vi "sub_psk_symbol_map_gen.vi"(9 "Gray code?":bool=TRUE, 11 "M-PSK":i32=4) -> (1 "index map":u32[](array[numeric]), 3 "symbol map":cdb[](array[numeric]))   [LabVIEW 2014]
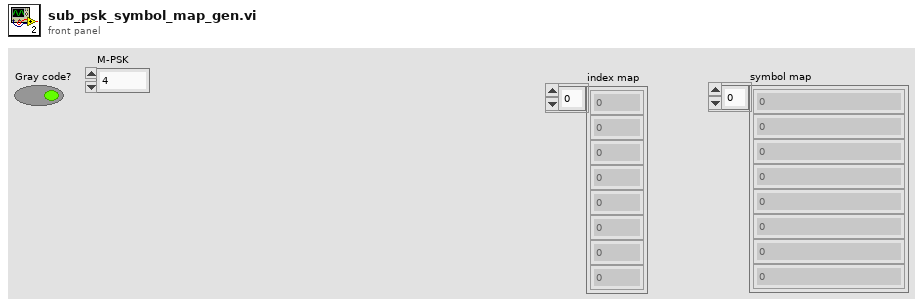
[diagram p1: front panel]
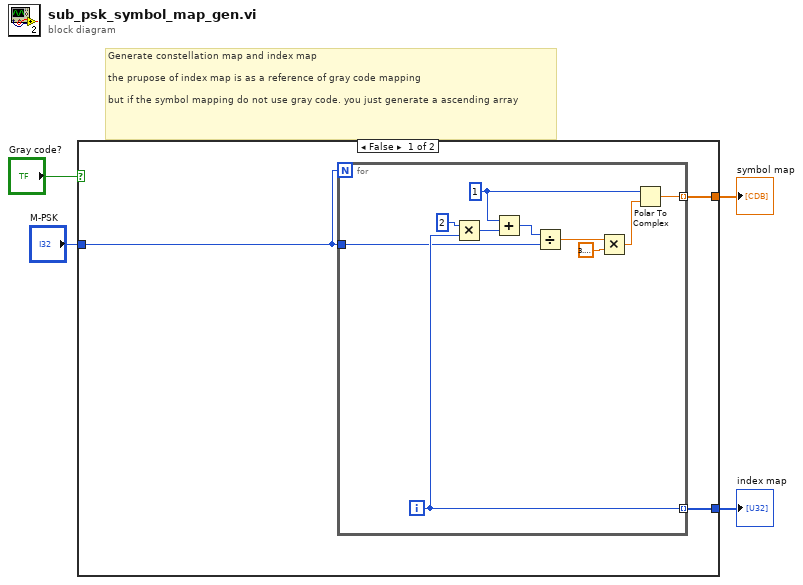
[diagram p0: block diagram]
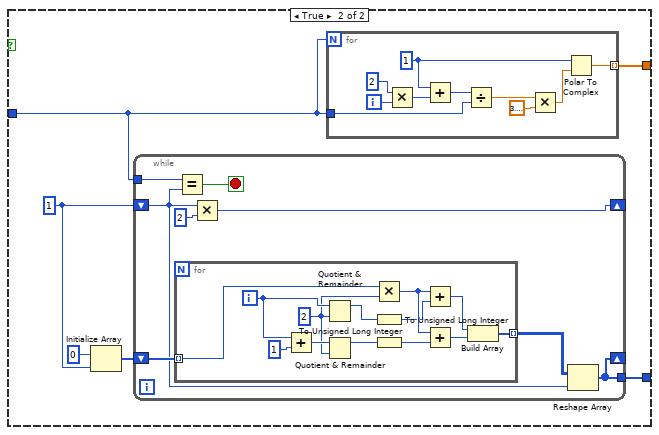
[diagram p2: hidden frame]
diagram:
  # "Generate constellation map and index map\n\nthe prupose of index map is as a reference of gray code mapping\n\nbut if the symbol mapping do not use gray code. you just generate a ascending array"
  n1 = case shown="False" "Gray code?" {
    tunnel: "M-PSK" -> [w6 w22]
    tunnel: [w7 w19] -> w2
    tunnel: [w5 w23] -> w1
    frame False {
      n2 = for {
        N: w6 -> [_]
        tunnel: [w17] -> w7 mode=indexing
        tunnel: w6 -> [w12]
        tunnel: [w8] -> w5 mode=indexing
        i -> [w17]
        w15 = 1
        n3 = Multiply(x=2, y=w17) -> (x*y=w14:i32)
        n4 = Add(x=w15, y=w14) -> (x+y=w13:i32)
        n5 = Divide(x=w13, y=w12) -> (x/y=w11:dbl)
        n6 = Multiply(x=w11, y=3.141592653589793) -> (x*y=w9:dbl)
        n7 = Polar To Complex(1:w9, 2:w15) -> (0:w8:cdb)
      }
    }
    frame True {
      w18 = u32 1
      n8 = Initialize Array(u32 0, w18) -> (w20:u32[])
      n9 = while {
        tunnel: w22 -> [w29]
        shift-right: [w31] -> _
        shift-left: w18 -> [w25]
        shift-right: [w24] -> _
        shift-left: w20 -> [w27]
        tunnel: [w24] -> w19
        stop <- w28 stop-if-true
        n10 = for {
          tunnel: w27 -> [w44] mode=indexing
          tunnel: [w34] -> w26 mode=indexing
          i -> [w43]
          w40 = u32 2
          n11 = Add(x=w43, y=u32 1) -> (x+y=w41:u32)
          n12 = Quotient & Remainder(x=w43, y=w40) -> (x-y*floor(x/y)=w33:u32)  [unwired: 1 out]
          n13 = Quotient & Remainder(x=w41, y=w40) -> (x-y*floor(x/y)=w32:u32)  [unwired: 1 out]
          n14 = Multiply(x=w44, y=w40) -> (x*y=w37:u32)
          n15 = To Unsigned Long Integer(number=w33) -> (unsigned 32bit integer=w36:u32)
          n16 = To Unsigned Long Integer(number=w32) -> (unsigned 32bit integer=w35:u32)
          n17 = Add(x=w37, y=w36) -> (x+y=w39:u32)
          n18 = Add(x=w37, y=w35) -> (x+y=w38:u32)
          n19 = Build Array(w39, w38) -> (w34:u32[])
        }
        n20 = Equal?(x=w29, y=w25) -> (x = y?=w28:bool)
        n21 = Multiply(x=w25, y=u32 2) -> (x*y=w31:u32)
        n22 = Reshape Array(w26, w25) -> (w24:u32[])
      }
      n23 = for {
        N: w22 -> [_]
        tunnel: w22 -> [w49]
        tunnel: [w45] -> w23 mode=indexing
        i -> [w54]
        w52 = 1
        n24 = Multiply(x=2, y=w54) -> (x*y=w51:i32)
        n25 = Add(x=w52, y=w51) -> (x+y=w50:i32)
        n26 = Divide(x=w50, y=w49) -> (x/y=w48:dbl)
        n27 = Multiply(x=w48, y=3.141592653589793) -> (x*y=w46:dbl)
        n28 = Polar To Complex(1:w46, 2:w52) -> (0:w45:cdb)
      }
    }
  }
  "symbol map" <- w1
  "index map" <- w2
